vi "refresh status.vi"(8 "error in (no error)":errorcluster, 10 "String In":string, 11 "Cascade in":refnum<class "Cascade.lvclass">) -> (0 "error out":errorcluster, 3 "Cascade out":refnum<class "Cascade.lvclass">)   [LabVIEW 2012, in "Cascade.lvclass"]
uses:
  Cascade.lvclass
  Cascade.lvclass/Cascade.ctl
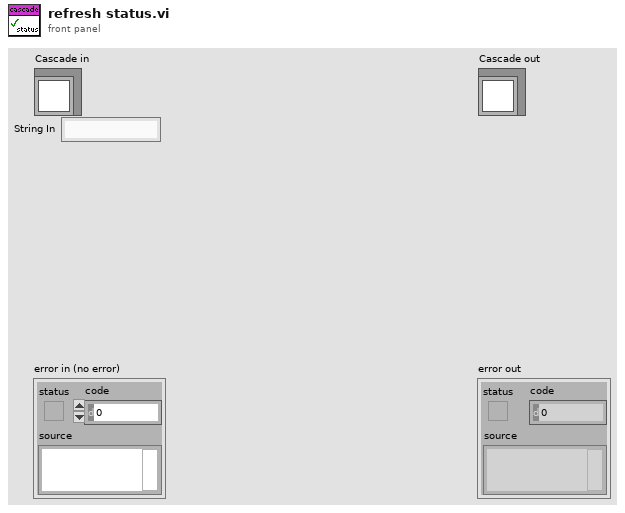
[diagram p1: front panel]
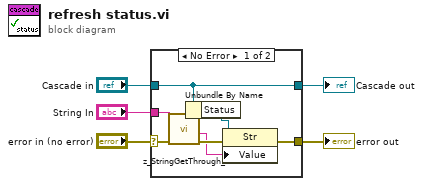
[diagram p0: block diagram]
diagram:
  n1 = case shown="No Error" "error in (no error)" {
    selector: "error in (no error)" -> [w12 w14]
    tunnel: [w9 w14] -> w4
    tunnel: [w11 w13] -> w2
    tunnel: "Cascade in" -> [w11 w13]
    tunnel: "String In" -> [w7 _]
    frame No Error {
      n2 = call "z_StringGetThrough_.vi"("Error In"=w12, "String In"=w7) -> ("Error Out"=w10:errorcluster, "String Out"=w6:string)  [unwired: 8 in]
      n3 = Unbundle By Name(w11) -> ("Status"=w8:refnum<vi>)
      n4 = property class="Str"(reference=w8, error in=w10, "Value"=w6) -> (error out=w9:errorcluster)  [unwired: 1 out]
    }
    frame Error {
    }
  }
  "error out" <- w4
  "Cascade out" <- w2
